vi "FillTest.vi"() -> ()   [LabVIEW 2016]
panel:
  in  "Reset Fill Amt":bool
  in  "Finish Filling":bool
  in  "Igniter Prime":bool
  in  "Fuel Prime":bool
  in  "Fill Rate (in^3/s)":dbl
  in  "Max Volume (in^3)":dbl
  in  "ARM":bool
  out "Fill Volume":dbl
  out "Fill Volume Bar":dbl(slide) max=258.9 scale=0.0..258.9
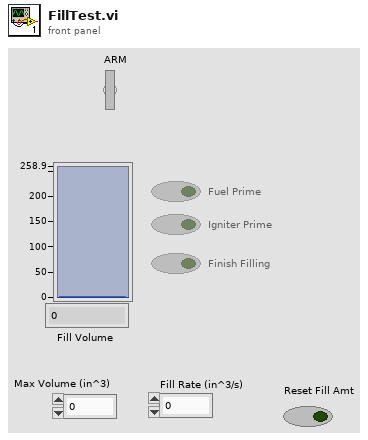
[diagram p1: front panel]
types:
  T1 = enum8{"Enabled", "Disabled", "Disabled and Grayed Out"}
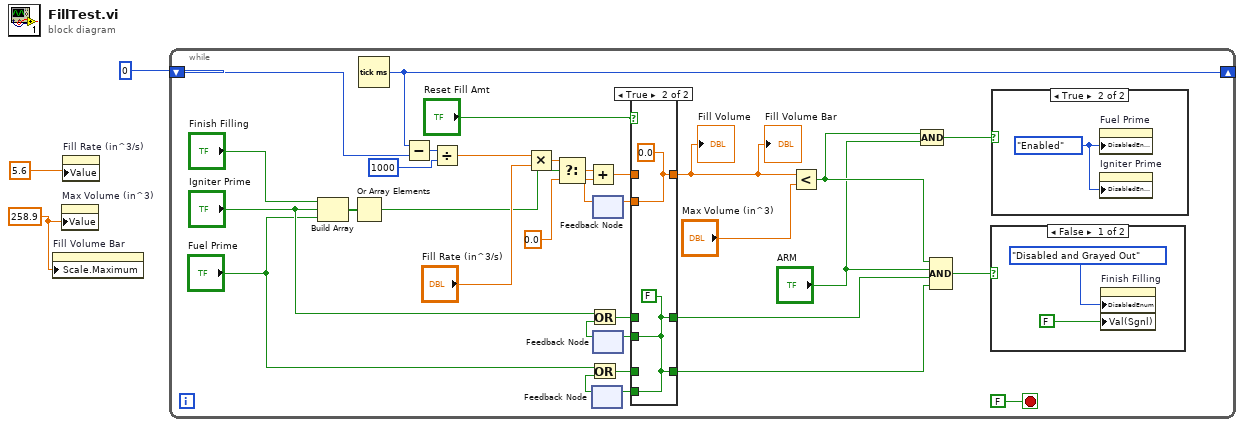
[diagram p0: block diagram]
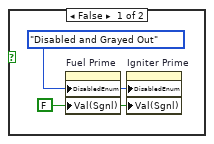
[diagram p3: hidden frame]
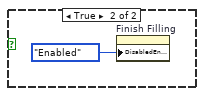
[diagram p4: hidden frame]
diagram:
  w1 = 258.9
  n1 = property on="Fill Volume Bar" class="Slide (strict)"("Scale.Maximum"=w1) -> ()  [unwired: 2 in, 2 out]
  n2 = property on="Max Volume (in^3)" class="DigNum (strict)"("Value"=w1) -> ()  [unwired: 2 in, 2 out]
  n3 = property on="Fill Rate (in^3/s)" class="DigNum (strict)"("Value"=5.6) -> ()  [unwired: 2 in, 2 out]
  n4 = while {
    shift-right: [w34] -> _
    shift-left: u32 0 ("millisecond timer value") -> [w35]
    stop <- FALSE stop-if-true
    n5 = Build Array("Finish Filling", "Igniter Prime", "Fuel Prime") -> (w24:bool[])
    n6 = Or Array Elements(Boolean array=w24) -> (logical OR=w25:bool)
    n7 = Tick Count (ms)() -> (millisecond timer value=w34:u32)
    n8 = Subtract(x=w34, y=w35) -> (x-y=w30:u32)
    n9 = Divide(x=w30, y=1000) -> (x/y=w29:dbl)
    n10 = Multiply(x=w29, y="Fill Rate (in^3/s)") -> (x*y=w33:dbl)
    n11 = Select(t=w33, s=w25, f=0.0) -> (s? t:f=w26:dbl)
    n12 = feedback #1() -> (w19:bool)  [unwired: 1 in]
    n13 = Or(x="Fuel Prime", y=w19) -> (x .or. y?=w17:bool)
    n14 = feedback #2() -> (w27:dbl)  [unwired: 1 in]
    n15 = Add(x=w26, y=w27) -> (x+y=w15:dbl)
    n16 = feedback #3() -> (w20:bool)  [unwired: 1 in]
    n17 = Or(x="Igniter Prime", y=w20) -> (x .or. y?=w16:bool)
    n18 = case shown="True" "Reset Fill Amt" {
      tunnel: w17 -> [w37 _]
      tunnel: w16 -> [w38 _]
      tunnel: w15 -> [w39 _]
      tunnel: [w39 w41] -> w14
      tunnel: [w39 w41] -> w13
      tunnel: [w38 w40] -> w8
      tunnel: [w38 w40] -> w12
      tunnel: [w37 w40] -> w7
      tunnel: [w37 w40] -> w11
      frame False {
      }
      frame True {
        w40 = FALSE
        w41 = 0.0
      }
    }
    "Fill Volume" <- w14
    "Fill Volume Bar" <- w14
    n19 = feedback-in #1(w11) -> ()
    n20 = feedback-in #2(w13) -> ()
    n21 = feedback-in #3(w12) -> ()
    n22 = Less?(x=w14, y="Max Volume (in^3)") -> (x < y?=w10:bool)
    n23 = Compound Arithmetic op=AND(w10, "ARM") -> (w23:bool)
    n24 = Compound Arithmetic op=AND(w10, "ARM", w8, w7) -> (w21:bool)
    n25 = case shown="False" w21 {
      frame False {
        n26 = property on="Finish Filling" class="Bool (strict)"("DisabledEnum"=T1."Disabled and Grayed Out" ("Disabled"), "Val(Sgnl)"=FALSE ("Value (Signaling)")) -> ()  [unwired: 2 in, 2 out]
      }
      frame True {
        n27 = property on="Finish Filling" class="Bool (strict)"("DisabledEnum"=T1."Enabled" ("Disabled")) -> ()  [unwired: 2 in, 2 out]
      }
    }
    n28 = case shown="True" w23 {
      frame False {
        w43 = T1."Disabled and Grayed Out" ("Disabled")
        w42 = FALSE ("Value (Signaling)")
        n29 = property on="Fuel Prime" class="Bool (strict)"("DisabledEnum"=w43, "Val(Sgnl)"=w42) -> ()  [unwired: 2 in, 2 out]
        n30 = property on="Igniter Prime" class="Bool (strict)"("DisabledEnum"=w43, "Val(Sgnl)"=w42) -> ()  [unwired: 2 in, 2 out]
      }
      frame True {
        w44 = T1."Enabled" ("Disabled")
        n31 = property on="Fuel Prime" class="Bool (strict)"("DisabledEnum"=w44) -> ()  [unwired: 2 in, 2 out]
        n32 = property on="Igniter Prime" class="Bool (strict)"("DisabledEnum"=w44) -> ()  [unwired: 2 in, 2 out]
      }
    }
  }
